vi "Matching String In Node Name.vi"(10 "Cluster":cluster{"Name":string, "Item Ref out":T1} {"Item Ref out" format="%.0x"}, 11 "Matching Strings":string[](array[string])) -> (3 "found?":bool)   [LabVIEW 2023, in "Protection and Counter Support System Explorer.lvlib"]
uses:
  Protection and Counter Support System Explorer.lvlib
  <vilib>/NI VeriStand/Custom Device API/Custom Device Item Ref.ctl
  <vilib>/NI VeriStand/Custom Device API/Custom Device API.lvlib
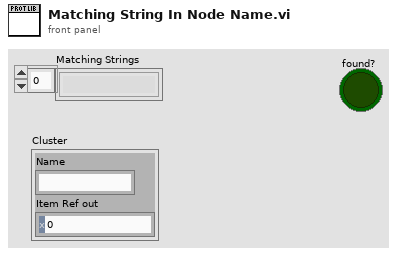
[diagram p1: front panel]
types:
  T1 = typedef "Custom Device API.lvlib/Custom Device Item Ref.ctl" = u64
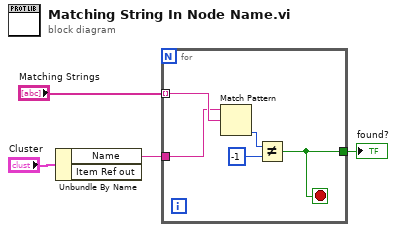
[diagram p0: block diagram]
diagram:
  n1 = Unbundle By Name("Cluster") -> ("Name"=w2:string)  [unwired: 1 out]
  n2 = for {
    tunnel: "Matching Strings" -> [w9] mode=indexing
    tunnel: w2 -> [w8]
    tunnel: [w5] -> w1
    stop <- w5 stop-if-true
    n3 = Match Pattern(string=w8, regular expression=w9) -> (offset past match=w7:i32)  [unwired: 1 in, 3 out]
    n4 = Not Equal?(x=w7, y=-1) -> (x != y?=w5:bool)
  }
  "found?" <- w1
